vi "DerivateActFuncArr.vi"(1 "Input":dbl[][](array[numeric])) -> (0 "Output":dbl[][](array[numeric]))   [LabVIEW 2021]
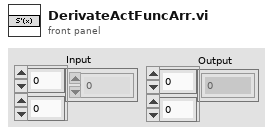
[diagram p1: front panel]
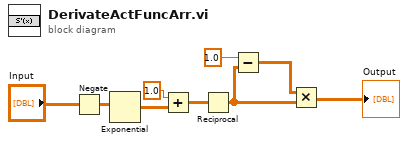
[diagram p0: block diagram]
diagram:
  n1 = Negate(x="Input") -> (-x=w9:dbl[][])
  n2 = Exponential(1:w9) -> (0:w7:dbl[][])
  n3 = Add(x=1.0, y=w7) -> (x+y=w6:dbl[][])
  n4 = Reciprocal(x=w6) -> (1/x=w3:dbl[][])
  n5 = Subtract(x=1.0, y=w3) -> (x-y=w4:dbl[][])
  n6 = Multiply(x=w4, y=w3) -> (x*y=→"Output":dbl[][])
